vi "输入数据解析.vi"(0 "单个参数补充":dbl, 1 "从板号":dbl=1.0, 2 "主板二维码":string="BNET01", 3 "从板二维码":string="BNET01", 5 "主板引用":refnum<vi>, 7 "从板引用":refnum<vi>, 9 "主板选项":string="三级故障阀值", 11 "枚举":enum16{"主板", "从板"}(ring), 12 "快换":bool caption="快换写入") -> (4 "输出数组":dbl[][](array[numeric]), 6 "数组长度":dbl[](array[numeric]), 8 "循环次数":i32, 10 "命令":u32, 14 "名称":string[](array[string]), 15 "命令序号":u32[](array[numeric]))   [LabVIEW 2013] (continued)
                    n3519 = call "输入分辨率计算-EV05.vi"("1字节?"=TRUE, "数值"=w9118, "偏移量"=-40.0, "分辨率"=1.0) -> ("高字节1"=w9121:dbl)  [unwired: 1 in, 6 out]
                  }
                  frame Enabled {
                  }
                }
                n3520 = Build Array(w9117) -> (w9116:i32[])
              }
              frame 4 {
                # "整组温度不均衡"
                n3521 = disable-structure shown="启用" {
                  disable-tunnel: [w9131 255 ("高字节1")] -> w9127
                  disable-tunnel: w9125 -> [w9129 _]
                  frame Disabled {
                    n3522 = Unbundle By Name(w9129) -> ("整组温度不均衡"=w9128:dbl)
                    n3523 = call "输入分辨率计算-EV05.vi"("1字节?"=TRUE, "数值"=w9128, "偏移量"=0.0, "分辨率"=1.0) -> ("高字节1"=w9131:dbl)  [unwired: 1 in, 6 out]
                  }
                  frame Enabled {
                  }
                }
                n3524 = Build Array(w9127) -> (w9126:i32[])
              }
              frame 5 {
                # "单组电压不均衡"
                n3525 = disable-structure shown="启用" {
                  disable-tunnel: [w9143 w9146] -> w9138
                  disable-tunnel: [w9141 w9146] -> w9136
                  disable-tunnel: w9135 -> [w9140 _]
                  frame Disabled {
                    n3526 = Unbundle By Name(w9140) -> ("单组电压不均衡"=w9139:dbl)
                    n3527 = call "输入分辨率计算-EV05.vi"("1字节?"=FALSE, "数值"=w9139, "偏移量"=0.0, "分辨率"=0.001) -> ("低字节"=w9141:dbl, "高字节1"=w9143:dbl)  [unwired: 1 in, 5 out]
                  }
                  frame Enabled {
                    w9146 = 255 ("高字节1")
                  }
                }
                n3528 = Build Array(w9138, w9136) -> (w9137:i32[])
              }
              frame 6 {
                # "整组电压不均衡"
                n3529 = disable-structure shown="启用" {
                  disable-tunnel: [w9155 w9158] -> w9150
                  disable-tunnel: [w9153 w9158] -> w9148
                  disable-tunnel: w9147 -> [w9152 _]
                  frame Disabled {
                    n3530 = Unbundle By Name(w9152) -> ("整组电压不均衡"=w9151:dbl)
                    n3531 = call "输入分辨率计算-EV05.vi"("1字节?"=FALSE, "数值"=w9151, "偏移量"=0.0, "分辨率"=0.001) -> ("低字节"=w9153:dbl, "高字节1"=w9155:dbl)  [unwired: 1 in, 5 out]
                  }
                  frame Enabled {
                    w9158 = 255 ("高字节1")
                  }
                }
                n3532 = Build Array(w9150, w9148) -> (w9149:i32[])
              }
              frame 7 {
                # "单体电压过高"
                n3533 = disable-structure shown="启用" {
                  disable-tunnel: [w9167 w9170] -> w9162
                  disable-tunnel: [w9165 w9170] -> w9160
                  disable-tunnel: w9159 -> [w9164 _]
                  frame Disabled {
                    n3534 = Unbundle By Name(w9164) -> ("单体电压过高"=w9163:dbl)
                    n3535 = call "输入分辨率计算-EV05.vi"("1字节?"=FALSE, "数值"=w9163, "偏移量"=0.0, "分辨率"=0.001) -> ("低字节"=w9165:dbl, "高字节1"=w9167:dbl)  [unwired: 1 in, 5 out]
                  }
                  frame Enabled {
                    w9170 = 255 ("高字节1")
                  }
                }
                n3536 = Build Array(w9162, w9160) -> (w9161:i32[])
              }
              frame 8 {
                # "单体电压过低"
                n3537 = disable-structure shown="启用" {
                  disable-tunnel: [w9179 w9182] -> w9174
                  disable-tunnel: [w9177 w9182] -> w9172
                  disable-tunnel: w9171 -> [w9176 _]
                  frame Disabled {
                    n3538 = Unbundle By Name(w9176) -> ("单体电压过低"=w9175:dbl)
                    n3539 = call "输入分辨率计算-EV05.vi"("1字节?"=FALSE, "数值"=w9175, "偏移量"=0.0, "分辨率"=0.001) -> ("低字节"=w9177:dbl, "高字节1"=w9179:dbl)  [unwired: 1 in, 5 out]
                  }
                  frame Enabled {
                    w9182 = 255 ("高字节1")
                  }
                }
                n3540 = Build Array(w9174, w9172) -> (w9173:i32[])
              }
              frame 9 {
                # "充电电流过高"
                n3541 = disable-structure shown="启用" {
                  disable-tunnel: [w9191 w9194] -> w9186
                  disable-tunnel: [w9189 w9194] -> w9184
                  disable-tunnel: w9183 -> [w9188 _]
                  frame Disabled {
                    n3542 = Unbundle By Name(w9188) -> ("充电电流过高"=w9187:dbl)
                    n3543 = call "输入分辨率计算-EV05.vi"("1字节?"=FALSE, "数值"=w9187, "偏移量"=-3000.0, "分辨率"=0.1) -> ("低字节"=w9189:dbl, "高字节1"=w9191:dbl)  [unwired: 1 in, 5 out]
                  }
                  frame Enabled {
                    w9194 = 255 ("高字节1")
                  }
                }
                n3544 = Build Array(w9186, w9184) -> (w9185:i32[])
              }
              frame 10 {
                # "放电电流过高"
                n3545 = disable-structure shown="启用" {
                  disable-tunnel: [w9203 w9206] -> w9198
                  disable-tunnel: [w9201 w9206] -> w9196
                  disable-tunnel: w9195 -> [w9200 _]
                  frame Disabled {
                    n3546 = Unbundle By Name(w9200) -> ("放电电流过高"=w9199:dbl)
                    n3547 = call "输入分辨率计算-EV05.vi"("1字节?"=FALSE, "数值"=w9199, "偏移量"=-3000.0, "分辨率"=0.1) -> ("低字节"=w9201:dbl, "高字节1"=w9203:dbl)  [unwired: 1 in, 5 out]
                  }
                  frame Enabled {
                    w9206 = 255 ("高字节1")
                  }
                }
                n3548 = Build Array(w9198, w9196) -> (w9197:i32[])
              }
              frame 11 {
                # "单组温度不均衡"
                n3549 = disable-structure shown="启用" {
                  disable-tunnel: [w9212 255 ("高字节1")] -> w9209
                  disable-tunnel: w9207 -> [w9211 _]
                  frame Enabled {
                    n3550 = Unbundle By Name(w9211) -> ("单组温度不均衡"=w9210:dbl)
                    n3551 = call "输入分辨率计算-EV05.vi"("1字节?"=TRUE, "数值"=w9210, "分辨率"=1.0) -> ("高字节1"=w9212:dbl)  [unwired: 2 in, 6 out]
                  }
                  frame Disabled {
                  }
                }
                n3552 = Build Array(w9209) -> (w9208:dbl[])
              }
              frame 12 {
                # "SOC过高"
                n3553 = Unbundle By Name(w9220) -> ("SOC过高"=w9219:dbl)
                n3554 = call "输入分辨率计算-EV05.vi"("1字节?"=FALSE, "数值"=w9219, "偏移量"=0.0, "分辨率"=0.1) -> ("低字节"=w9221:dbl, "高字节1"=w9222:dbl)  [unwired: 1 in, 5 out]
                n3555 = call "二进制解析-8.6.vi"("索引"=4, "数值"=w9222) -> ("低位子数组"=w9225:i32[])  [unwired: 3 out]
                n3556 = call "二进制解析-8.6.vi"("索引"=4, "数值"=w9221) -> ("低位子数组"=w9217:i32[], "高位子数组"=w9224:i32[])  [unwired: 2 out]
                n3557 = Insert Into Array(array=w9225, new element=w9224) -> (w9223:i32[])  [unwired: 1 in]
                n3558 = call "数值二进制转十进制-8.6.vi"("子数组"=w9223) -> ("十进制数值"=w9218:i32)  [unwired: 4 out]
                n3559 = disable-structure shown="启用" {
                  disable-tunnel: w9218 -> [w9233 _]
                  disable-tunnel: [w9233 255 ("高字节1")] -> w9216
                  disable-tunnel: w9217 -> [w9232 _]
                  disable-tunnel: [w9232 i32[] [] ("低位子数组 29")] -> _
                  frame Disabled {
                  }
                  frame Enabled {
                  }
                }
                n3560 = Build Array(w9216, w9216) -> (w9229:i32[])
              }
              frame 13 {
                # "SOC过低"
                n3561 = Unbundle By Name(w9241) -> ("SOC过低"=w9240:dbl)
                n3562 = call "输入分辨率计算-EV05.vi"("1字节?"=FALSE, "数值"=w9240, "偏移量"=0.0, "分辨率"=0.1) -> ("低字节"=w9238:dbl, "高字节1"=w9239:dbl)  [unwired: 1 in, 5 out]
                n3563 = call "二进制解析-8.6.vi"("索引"=4, "数值"=w9239) -> ("低位子数组"=w9237:i32[])  [unwired: 3 out]
                n3564 = disable-structure shown="启用" {
                  disable-tunnel: w9238 -> [w9248 _]
                  disable-tunnel: [w9248 255 ("高字节1")] -> w9236
                  disable-tunnel: w9237 -> [w9247 _]
                  disable-tunnel: [w9247 i32[] [] ("低位子数组")] -> _
                  frame Disabled {
                    (unwired) i32[] [] ("低位子数组 4")
                  }
                  frame Enabled {
                  }
                }
                n3565 = Build Array(w9236, w9236) -> (w9244:i32[])
              }
              frame 14 {
                # "内阻过大"
                n3566 = disable-structure shown="启用" {
                  disable-tunnel: w9253 -> [w9258 _]
                  disable-tunnel: [w9254 255 ("高字节1")] -> w9251
                  frame Disabled {
                    n3567 = Unbundle By Name(w9258) -> ("内阻过大"=w9257:dbl)
                    n3568 = call "输入分辨率计算-EV05.vi"("1字节?"=TRUE, "数值"=w9257, "分辨率"=0.1) -> ("高字节1"=w9254:dbl)  [unwired: 2 in, 6 out]
                  }
                  frame Enabled {
                  }
                }
                n3569 = Build Array(w9251) -> (w9252:i32[])
              }
              frame 15 {
                # "极柱温度过高"
                n3570 = disable-structure shown="启用" {
                  disable-tunnel: w9262 -> [w9268 _]
                  disable-tunnel: [w9264 255 ("高字节1")] -> w9260
                  frame Disabled {
                    n3571 = Unbundle By Name(w9268) -> ("极柱温度过高"=w9267:dbl)
                    n3572 = call "输入分辨率计算-EV05.vi"("1字节?"=TRUE, "数值"=w9267, "偏移量"=-40.0, "分辨率"=1.0) -> ("高字节1"=w9264:dbl)  [unwired: 1 in, 6 out]
                  }
                  frame Enabled {
                  }
                }
                n3573 = Build Array(w9260) -> (w9261:i32[])
              }
              frame 16 {
                # "SOH过低"
                n3574 = disable-structure shown="启用" {
                  disable-tunnel: [w9285 w9293] -> w9272
                  disable-tunnel: w9271 -> [w9282 _]
                  disable-tunnel: [w9274 w9293] -> w9270
                  frame Disabled {
                    n3575 = Unbundle By Name(w9282) -> ("SOH过低"=w9281:dbl)
                    n3576 = call "输入分辨率计算-EV05.vi"("1字节?"=FALSE, "数值"=w9281, "偏移量"=0.0, "分辨率"=0.1) -> ("低字节"=w9283:dbl, "高字节1"=w9284:dbl)  [unwired: 1 in, 5 out]
                    n3577 = call "二进制解析-8.6.vi"("索引"=4, "数值"=w9284) -> ("低位子数组"=w9287:i32[])  [unwired: 3 out]
                    n3578 = call "二进制解析-8.6.vi"("索引"=4, "数值"=w9283) -> ("低位子数组"=w9276:i32[], "高位子数组"=w9286:i32[])  [unwired: 2 out]
                    n3579 = call "二进制解析-8.6.vi"("索引"=4, "数值"=0) -> ("低位子数组"=w9277:i32[])  [unwired: 3 out]
                    n3580 = Insert Into Array(array=w9287, new element=w9286) -> (w9280:i32[])  [unwired: 1 in]
                    n3581 = Insert Into Array(array=w9276, new element=w9277) -> (w9275:i32[])  [unwired: 1 in]
                    n3582 = call "数值二进制转十进制-8.6.vi"("子数组"=w9280) -> ("十进制数值"=w9285:i32)  [unwired: 4 out]
                    n3583 = call "数值二进制转十进制-8.6.vi"("子数组"=w9275) -> ("十进制数值"=w9274:i32)  [unwired: 4 out]
                  }
                  frame Enabled {
                    w9293 = 255 ("高字节1")
                  }
                }
                n3584 = Build Array(w9272, w9270) -> (w9273:i32[])
              }
            }
            n3585 = Insert Into Array(array=w9079, new element=w9080) -> (w9078:dbl[])  [unwired: 1 in]
          }
          n3586 = Build Array(w9075) -> (w9074:dbl[][])
          n3587 = Build Array("三级故障阀值") -> (w9065:string[])
        }
        frame "内阻过大" {
          n3588 = Unbundle By Name(w9299) -> ("一级故障"=w9300:refnum<vi>)
          n3589 = property class="Clust (严格)"(reference=w9300) -> ("Value"=w9298:T4)  [unwired: 1 in, 2 out]
          n3590 = for {
            N: 17 -> [_]
            tunnel: w9298 -> [w9310]
            shift-right: [w9307] -> w9304
            shift-left: dbl[] [] -> [w9308]
            i -> [w9311]
            n3591 = case shown="13" w9311 {
              tunnel: w9310 -> [w9312 w9323 w9334 w9344 w9354 w9364 w9376 w9388 w9400 w9412 w9424 w9436 w9450 w9471 w9483 w9492 w9501]
              tunnel: [w9313 w9324 w9335 w9345 w9355 w9366 w9378 w9390 w9402 w9414 w9426 w9437 w9459 w9474 w9482 w9491 w9503] -> w9309
              frame 0, Default {
                # "总电压过高"
                n3592 = disable-structure shown="启用" {
                  disable-tunnel: [w9319 w9322] -> w9315
                  disable-tunnel: [w9318 w9322] -> w9314
                  disable-tunnel: w9312 -> [w9317 _]
                  frame Disabled {
                    n3593 = Unbundle By Name(w9317) -> ("总电压过高"=w9316:dbl)
                    n3594 = call "输入分辨率计算-EV05.vi"("1字节?"=FALSE, "数值"=w9316, "分辨率"=0.1) -> ("低字节"=w9319:dbl, "高字节1"=w9318:dbl)  [unwired: 2 in, 5 out]
                  }
                  frame Enabled {
                    w9322 = 255 ("高字节1")
                  }
                }
                n3595 = Build Array(w9314, w9315) -> (w9313:i32[])
              }
              frame 1 {
                # "总电压过低"
                n3596 = disable-structure shown="启用" {
                  disable-tunnel: [w9330 w9333] -> w9326
                  disable-tunnel: [w9329 w9333] -> w9325
                  disable-tunnel: w9323 -> [w9328 _]
                  frame Disabled {
                    n3597 = Unbundle By Name(w9328) -> ("总电压过低"=w9327:dbl)
                    n3598 = call "输入分辨率计算-EV05.vi"("1字节?"=FALSE, "数值"=w9327, "分辨率"=0.1) -> ("低字节"=w9330:dbl, "高字节1"=w9329:dbl)  [unwired: 2 in, 5 out]
                  }
                  frame Enabled {
                    w9333 = 255 ("高字节1")
                  }
                }
                n3599 = Build Array(w9325, w9326) -> (w9324:i32[])
              }
              frame 2 {
                # "温度过高"
                n3600 = disable-structure shown="启用" {
                  disable-tunnel: [w9340 255 ("高字节1")] -> w9336
                  disable-tunnel: w9334 -> [w9338 _]
                  frame Disabled {
                    n3601 = Unbundle By Name(w9338) -> ("温度过高"=w9337:dbl)
                    n3602 = call "输入分辨率计算-EV05.vi"("1字节?"=TRUE, "数值"=w9337, "偏移量"=-40.0, "分辨率"=1.0) -> ("高字节1"=w9340:dbl)  [unwired: 1 in, 6 out]
                  }
                  frame Enabled {
                  }
                }
                n3603 = Build Array(w9336) -> (w9335:i32[])
              }
              frame 3 {
                # "温度过低"
                n3604 = disable-structure shown="启用" {
                  disable-tunnel: [w9350 255 ("高字节1")] -> w9346
                  disable-tunnel: w9344 -> [w9348 _]
                  frame Disabled {
                    n3605 = Unbundle By Name(w9348) -> ("温度过低"=w9347:dbl)
                    n3606 = call "输入分辨率计算-EV05.vi"("1字节?"=TRUE, "数值"=w9347, "偏移量"=-40.0, "分辨率"=1.0) -> ("高字节1"=w9350:dbl)  [unwired: 1 in, 6 out]
                  }
                  frame Enabled {
                  }
                }
                n3607 = Build Array(w9346) -> (w9345:i32[])
              }
              frame 4 {
                # "整组温度不均衡"
                n3608 = disable-structure shown="启用" {
                  disable-tunnel: [w9360 255 ("高字节1")] -> w9356
                  disable-tunnel: w9354 -> [w9358 _]
                  frame Disabled {
                    n3609 = Unbundle By Name(w9358) -> ("整组温度不均衡"=w9357:dbl)
                    n3610 = call "输入分辨率计算-EV05.vi"("1字节?"=TRUE, "数值"=w9357, "偏移量"=0.0, "分辨率"=1.0) -> ("高字节1"=w9360:dbl)  [unwired: 1 in, 6 out]
                  }
                  frame Enabled {
                  }
                }
                n3611 = Build Array(w9356) -> (w9355:i32[])
              }
              frame 5 {
                # "单组电压不均衡"
                n3612 = disable-structure shown="启用" {
                  disable-tunnel: [w9372 w9375] -> w9367
                  disable-tunnel: [w9370 w9375] -> w9365
                  disable-tunnel: w9364 -> [w9369 _]
                  frame Disabled {
                    n3613 = Unbundle By Name(w9369) -> ("单组电压不均衡"=w9368:dbl)
                    n3614 = call "输入分辨率计算-EV05.vi"("1字节?"=FALSE, "数值"=w9368, "偏移量"=0.0, "分辨率"=0.001) -> ("低字节"=w9370:dbl, "高字节1"=w9372:dbl)  [unwired: 1 in, 5 out]
                  }
                  frame Enabled {
                    w9375 = 255 ("高字节1")
                  }
                }
                n3615 = Build Array(w9367, w9365) -> (w9366:i32[])
              }
              frame 6 {
                # "整组电压不均衡"
                n3616 = disable-structure shown="启用" {
                  disable-tunnel: [w9384 w9387] -> w9379
                  disable-tunnel: [w9382 w9387] -> w9377
                  disable-tunnel: w9376 -> [w9381 _]
                  frame Disabled {
                    n3617 = Unbundle By Name(w9381) -> ("整组电压不均衡"=w9380:dbl)
                    n3618 = call "输入分辨率计算-EV05.vi"("1字节?"=FALSE, "数值"=w9380, "偏移量"=0.0, "分辨率"=0.001) -> ("低字节"=w9382:dbl, "高字节1"=w9384:dbl)  [unwired: 1 in, 5 out]
                  }
                  frame Enabled {
                    w9387 = 255 ("高字节1")
                  }
                }
                n3619 = Build Array(w9379, w9377) -> (w9378:i32[])
              }
              frame 7 {
                # "单体电压过高"
                n3620 = disable-structure shown="启用" {
                  disable-tunnel: [w9396 w9399] -> w9391
                  disable-tunnel: [w9394 w9399] -> w9389
                  disable-tunnel: w9388 -> [w9393 _]
                  frame Disabled {
                    n3621 = Unbundle By Name(w9393) -> ("单体电压过高"=w9392:dbl)
                    n3622 = call "输入分辨率计算-EV05.vi"("1字节?"=FALSE, "数值"=w9392, "偏移量"=0.0, "分辨率"=0.001) -> ("低字节"=w9394:dbl, "高字节1"=w9396:dbl)  [unwired: 1 in, 5 out]
                  }
                  frame Enabled {
                    w9399 = 255 ("高字节1")
                  }
                }
                n3623 = Build Array(w9391, w9389) -> (w9390:i32[])
              }
              frame 8 {
                # "单体电压过低"
                n3624 = disable-structure shown="启用" {
                  disable-tunnel: [w9408 w9411] -> w9403
                  disable-tunnel: [w9406 w9411] -> w9401
                  disable-tunnel: w9400 -> [w9405 _]
                  frame Disabled {
                    n3625 = Unbundle By Name(w9405) -> ("单体电压过低"=w9404:dbl)
                    n3626 = call "输入分辨率计算-EV05.vi"("1字节?"=FALSE, "数值"=w9404, "偏移量"=0.0, "分辨率"=0.001) -> ("低字节"=w9406:dbl, "高字节1"=w9408:dbl)  [unwired: 1 in, 5 out]
                  }
                  frame Enabled {
                    w9411 = 255 ("高字节1")
                  }
                }
                n3627 = Build Array(w9403, w9401) -> (w9402:i32[])
              }
              frame 9 {
                # "充电电流过高"
                n3628 = disable-structure shown="启用" {
                  disable-tunnel: [w9420 w9423] -> w9415
                  disable-tunnel: [w9418 w9423] -> w9413
                  disable-tunnel: w9412 -> [w9417 _]
                  frame Disabled {
                    n3629 = Unbundle By Name(w9417) -> ("充电电流过高"=w9416:dbl)
                    n3630 = call "输入分辨率计算-EV05.vi"("1字节?"=FALSE, "数值"=w9416, "偏移量"=-3000.0, "分辨率"=0.1) -> ("低字节"=w9418:dbl, "高字节1"=w9420:dbl)  [unwired: 1 in, 5 out]
                  }
                  frame Enabled {
                    w9423 = 255 ("高字节1")
                  }
                }
                n3631 = Build Array(w9415, w9413) -> (w9414:i32[])
              }
              frame 10 {
                # "放电电流过高"
                n3632 = disable-structure shown="启用" {
                  disable-tunnel: [w9432 w9435] -> w9427
                  disable-tunnel: [w9430 w9435] -> w9425
                  disable-tunnel: w9424 -> [w9429 _]
                  frame Disabled {
                    n3633 = Unbundle By Name(w9429) -> ("放电电流过高"=w9428:dbl)
                    n3634 = call "输入分辨率计算-EV05.vi"("1字节?"=FALSE, "数值"=w9428, "偏移量"=-3000.0, "分辨率"=0.1) -> ("低字节"=w9430:dbl, "高字节1"=w9432:dbl)  [unwired: 1 in, 5 out]
                  }
                  frame Enabled {
                    w9435 = 255 ("高字节1")
                  }
                }
                n3635 = Build Array(w9427, w9425) -> (w9426:i32[])
              }
              frame 11 {
                # "单组温度不均衡"
                n3636 = disable-structure shown="启用" {
                  disable-tunnel: [w9442 255 ("高字节1")] -> w9438
                  disable-tunnel: w9436 -> [w9440 _]
                  frame Disabled {
                    n3637 = Unbundle By Name(w9440) -> ("单组温度不均衡"=w9439:dbl)
                    n3638 = call "输入分辨率计算-EV05.vi"("1字节?"=TRUE, "数值"=w9439, "偏移量"=0.0, "分辨率"=1.0) -> ("高字节1"=w9442:dbl)  [unwired: 1 in, 6 out]
                  }
                  frame Enabled {
                  }
                }
                n3639 = Build Array(w9438) -> (w9437:i32[])
              }
              frame 12 {
                # "SOC过高"
                n3640 = Unbundle By Name(w9450) -> ("SOC过高"=w9449:dbl)
                n3641 = call "输入分辨率计算-EV05.vi"("1字节?"=FALSE, "数值"=w9449, "偏移量"=0.0, "分辨率"=0.1) -> ("低字节"=w9451:dbl, "高字节1"=w9452:dbl)  [unwired: 1 in, 5 out]
                n3642 = call "二进制解析-8.6.vi"("索引"=4, "数值"=w9452) -> ("低位子数组"=w9455:i32[])  [unwired: 3 out]
                n3643 = call "二进制解析-8.6.vi"("索引"=4, "数值"=w9451) -> ("低位子数组"=w9447:i32[], "高位子数组"=w9454:i32[])  [unwired: 2 out]
                n3644 = Insert Into Array(array=w9455, new element=w9454) -> (w9453:i32[])  [unwired: 1 in]
                n3645 = call "数值二进制转十进制-8.6.vi"("子数组"=w9453) -> ("十进制数值"=w9448:i32)  [unwired: 4 out]
                n3646 = disable-structure shown="启用" {
                  disable-tunnel: w9448 -> [w9463 _]
                  disable-tunnel: [w9463 255 ("高字节1")] -> w9446
                  disable-tunnel: w9447 -> [w9462 _]
                  disable-tunnel: [w9462 i32[] [] ("低位子数组 29")] -> _
                  frame Disabled {
                  }
                  frame Enabled {
                  }
                }
                n3647 = Build Array(w9446, w9446) -> (w9459:i32[])
              }
              frame 13 {
                # "SOC过低"
                n3648 = Unbundle By Name(w9471) -> ("SOC过低"=w9470:dbl)
                n3649 = call "输入分辨率计算-EV05.vi"("1字节?"=FALSE, "数值"=w9470, "偏移量"=0.0, "分辨率"=0.1) -> ("低字节"=w9468:dbl, "高字节1"=w9469:dbl)  [unwired: 1 in, 5 out]
                n3650 = call "二进制解析-8.6.vi"("索引"=4, "数值"=w9469) -> ("低位子数组"=w9467:i32[])  [unwired: 3 out]
                n3651 = disable-structure shown="启用" {
                  disable-tunnel: w9468 -> [w9478 _]
                  disable-tunnel: [w9478 255 ("高字节1")] -> w9466
                  disable-tunnel: w9467 -> [w9477 _]
                  disable-tunnel: [w9477 i32[] [] ("低位子数组")] -> _
                  frame Disabled {
                    (unwired) i32[] [] ("低位子数组 4")
                  }
                  frame Enabled {
                  }
                }
                n3652 = Build Array(w9466, w9466) -> (w9474:i32[])
              }
              frame 14 {
                # "内阻过大"
                n3653 = disable-structure shown="启用" {
                  disable-tunnel: w9483 -> [w9488 _]
                  disable-tunnel: [w9484 255 ("高字节1")] -> w9481
                  frame Enabled {
                    n3654 = Unbundle By Name(w9488) -> ("内阻过大"=w9487:dbl)
                    n3655 = call "输入分辨率计算-EV05.vi"("1字节?"=TRUE, "数值"=w9487, "分辨率"=0.1) -> ("高字节1"=w9484:dbl)  [unwired: 2 in, 6 out]
                  }
                  frame Disabled {
                  }
                }
                n3656 = Build Array(w9481) -> (w9482:dbl[])
              }
              frame 15 {
                # "极柱温度过高"
                n3657 = disable-structure shown="启用" {
                  disable-tunnel: w9492 -> [w9498 _]
                  disable-tunnel: [w9494 255 ("高字节1")] -> w9490
                  frame Disabled {
                    n3658 = Unbundle By Name(w9498) -> ("极柱温度过高"=w9497:dbl)
                    n3659 = call "输入分辨率计算-EV05.vi"("1字节?"=TRUE, "数值"=w9497, "偏移量"=-40.0, "分辨率"=1.0) -> ("高字节1"=w9494:dbl)  [unwired: 1 in, 6 out]
                  }
                  frame Enabled {
                  }
                }
                n3660 = Build Array(w9490) -> (w9491:i32[])
              }
              frame 16 {
                # "SOH过低"
                n3661 = disable-structure shown="启用" {
                  disable-tunnel: [w9515 w9523] -> w9502
                  disable-tunnel: w9501 -> [w9512 _]
                  disable-tunnel: [w9504 w9523] -> w9500
                  frame Disabled {
                    n3662 = Unbundle By Name(w9512) -> ("SOH过低"=w9511:dbl)
                    n3663 = call "输入分辨率计算-EV05.vi"("1字节?"=FALSE, "数值"=w9511, "偏移量"=0.0, "分辨率"=0.1) -> ("低字节"=w9513:dbl, "高字节1"=w9514:dbl)  [unwired: 1 in, 5 out]
                    n3664 = call "二进制解析-8.6.vi"("索引"=4, "数值"=w9514) -> ("低位子数组"=w9517:i32[])  [unwired: 3 out]
                    n3665 = call "二进制解析-8.6.vi"("索引"=4, "数值"=w9513) -> ("低位子数组"=w9506:i32[], "高位子数组"=w9516:i32[])  [unwired: 2 out]
                    n3666 = call "二进制解析-8.6.vi"("索引"=4, "数值"=0) -> ("低位子数组"=w9507:i32[])  [unwired: 3 out]
                    n3667 = Insert Into Array(array=w9517, new element=w9516) -> (w9510:i32[])  [unwired: 1 in]
                    n3668 = Insert Into Array(array=w9506, new element=w9507) -> (w9505:i32[])  [unwired: 1 in]
                    n3669 = call "数值二进制转十进制-8.6.vi"("子数组"=w9510) -> ("十进制数值"=w9515:i32)  [unwired: 4 out]
                    n3670 = call "数值二进制转十进制-8.6.vi"("子数组"=w9505) -> ("十进制数值"=w9504:i32)  [unwired: 4 out]
                  }
                  frame Enabled {
                    w9523 = 255 ("高字节1")
                  }
                }
                n3671 = Build Array(w9502, w9500) -> (w9503:i32[])
              }
            }
            n3672 = Insert Into Array(array=w9308, new element=w9309) -> (w9307:dbl[])  [unwired: 1 in]
          }
          n3673 = Build Array(w9304) -> (w9303:dbl[][])
          n3674 = Build Array("一级故障阀值") -> (w9294:string[])
        }
        frame "内阻过大(2)" {
          n3675 = Unbundle By Name(w9529) -> ("一级故障 2"=w9530:refnum<vi>)
          n3676 = property class="Clust (严格)"(reference=w9530) -> ("Value"=w9528:T4)  [unwired: 1 in, 2 out]
          n3677 = for {
            N: 17 -> [_]
            tunnel: w9528 -> [w9540]
            shift-right: [w9537] -> w9534
            shift-left: dbl[] [] -> [w9538]
            i -> [w9541]
            n3678 = case shown="13" w9541 {
              tunnel: w9540 -> [w9542 w9553 w9564 w9574 w9584 w9594 w9606 w9618 w9630 w9642 w9654 w9666 w9680 w9701 w9713 w9722 w9731]
              tunnel: [w9543 w9554 w9565 w9575 w9585 w9596 w9608 w9620 w9632 w9644 w9656 w9667 w9689 w9704 w9712 w9721 w9733] -> w9539
              frame 0, Default {
                # "总电压过高"
                n3679 = disable-structure shown="启用" {
                  disable-tunnel: [w9549 w9552] -> w9545
                  disable-tunnel: [w9548 w9552] -> w9544
                  disable-tunnel: w9542 -> [w9547 _]
                  frame Disabled {
                    n3680 = Unbundle By Name(w9547) -> ("总电压过高"=w9546:dbl)
                    n3681 = call "输入分辨率计算-EV05.vi"("1字节?"=FALSE, "数值"=w9546, "分辨率"=0.1) -> ("低字节"=w9549:dbl, "高字节1"=w9548:dbl)  [unwired: 2 in, 5 out]
                  }
                  frame Enabled {
                    w9552 = 255 ("高字节1")
                  }
                }
                n3682 = Build Array(w9544, w9545) -> (w9543:i32[])
              }
              frame 1 {
                # "总电压过低"
                n3683 = disable-structure shown="启用" {
                  disable-tunnel: [w9560 w9563] -> w9556
                  disable-tunnel: [w9559 w9563] -> w9555
                  disable-tunnel: w9553 -> [w9558 _]
                  frame Disabled {
                    n3684 = Unbundle By Name(w9558) -> ("总电压过低"=w9557:dbl)
                    n3685 = call "输入分辨率计算-EV05.vi"("1字节?"=FALSE, "数值"=w9557, "分辨率"=0.1) -> ("低字节"=w9560:dbl, "高字节1"=w9559:dbl)  [unwired: 2 in, 5 out]
                  }
                  frame Enabled {
                    w9563 = 255 ("高字节1")
                  }
                }
                n3686 = Build Array(w9555, w9556) -> (w9554:i32[])
              }
              frame 2 {
                # "温度过高"
                n3687 = disable-structure shown="启用" {
                  disable-tunnel: [w9570 255 ("高字节1")] -> w9566
                  disable-tunnel: w9564 -> [w9568 _]
                  frame Disabled {
                    n3688 = Unbundle By Name(w9568) -> ("温度过高"=w9567:dbl)
                    n3689 = call "输入分辨率计算-EV05.vi"("1字节?"=TRUE, "数值"=w9567, "偏移量"=-40.0, "分辨率"=1.0) -> ("高字节1"=w9570:dbl)  [unwired: 1 in, 6 out]
                  }
                  frame Enabled {
                  }
                }
                n3690 = Build Array(w9566) -> (w9565:i32[])
              }
              frame 3 {
                # "温度过低"
                n3691 = disable-structure shown="启用" {
                  disable-tunnel: [w9580 255 ("高字节1")] -> w9576
                  disable-tunnel: w9574 -> [w9578 _]
                  frame Disabled {
                    n3692 = Unbundle By Name(w9578) -> ("温度过低"=w9577:dbl)
                    n3693 = call "输入分辨率计算-EV05.vi"("1字节?"=TRUE, "数值"=w9577, "偏移量"=-40.0, "分辨率"=1.0) -> ("高字节1"=w9580:dbl)  [unwired: 1 in, 6 out]
                  }
                  frame Enabled {
                  }
                }
                n3694 = Build Array(w9576) -> (w9575:i32[])
              }
              frame 4 {
                # "整组温度不均衡"
                n3695 = disable-structure shown="启用" {
                  disable-tunnel: [w9590 255 ("高字节1")] -> w9586
                  disable-tunnel: w9584 -> [w9588 _]
                  frame Disabled {
                    n3696 = Unbundle By Name(w9588) -> ("整组温度不均衡"=w9587:dbl)
                    n3697 = call "输入分辨率计算-EV05.vi"("1字节?"=TRUE, "数值"=w9587, "偏移量"=0.0, "分辨率"=1.0) -> ("高字节1"=w9590:dbl)  [unwired: 1 in, 6 out]
                  }
                  frame Enabled {
                  }
                }
                n3698 = Build Array(w9586) -> (w9585:i32[])
              }
              frame 5 {
                # "单组电压不均衡"
                n3699 = disable-structure shown="启用" {
                  disable-tunnel: [w9602 w9605] -> w9597
                  disable-tunnel: [w9600 w9605] -> w9595
                  disable-tunnel: w9594 -> [w9599 _]
                  frame Disabled {
                    n3700 = Unbundle By Name(w9599) -> ("单组电压不均衡"=w9598:dbl)
                    n3701 = call "输入分辨率计算-EV05.vi"("1字节?"=FALSE, "数值"=w9598, "偏移量"=0.0, "分辨率"=0.001) -> ("低字节"=w9600:dbl, "高字节1"=w9602:dbl)  [unwired: 1 in, 5 out]
                  }
                  frame Enabled {
                    w9605 = 255 ("高字节1")
                  }
                }
                n3702 = Build Array(w9597, w9595) -> (w9596:i32[])
              }
              frame 6 {
                # "整组电压不均衡"
                n3703 = disable-structure shown="启用" {
                  disable-tunnel: [w9614 w9617] -> w9609
                  disable-tunnel: [w9612 w9617] -> w9607
                  disable-tunnel: w9606 -> [w9611 _]
                  frame Disabled {
                    n3704 = Unbundle By Name(w9611) -> ("整组电压不均衡"=w9610:dbl)
                    n3705 = call "输入分辨率计算-EV05.vi"("1字节?"=FALSE, "数值"=w9610, "偏移量"=0.0, "分辨率"=0.001) -> ("低字节"=w9612:dbl, "高字节1"=w9614:dbl)  [unwired: 1 in, 5 out]
                  }
                  frame Enabled {
                    w9617 = 255 ("高字节1")
                  }
                }
                n3706 = Build Array(w9609, w9607) -> (w9608:i32[])
              }
              frame 7 {
                # "单体电压过高"
                n3707 = disable-structure shown="启用" {
                  disable-tunnel: [w9626 w9629] -> w9621
                  disable-tunnel: [w9624 w9629] -> w9619
                  disable-tunnel: w9618 -> [w9623 _]
                  frame Disabled {
                    n3708 = Unbundle By Name(w9623) -> ("单体电压过高"=w9622:dbl)
                    n3709 = call "输入分辨率计算-EV05.vi"("1字节?"=FALSE, "数值"=w9622, "偏移量"=0.0, "分辨率"=0.001) -> ("低字节"=w9624:dbl, "高字节1"=w9626:dbl)  [unwired: 1 in, 5 out]
                  }
                  frame Enabled {
                    w9629 = 255 ("高字节1")
                  }
                }
                n3710 = Build Array(w9621, w9619) -> (w9620:i32[])
              }
              frame 8 {
                # "单体电压过低"
                n3711 = disable-structure shown="启用" {
                  disable-tunnel: [w9638 w9641] -> w9633
                  disable-tunnel: [w9636 w9641] -> w9631
                  disable-tunnel: w9630 -> [w9635 _]
                  frame Disabled {
                    n3712 = Unbundle By Name(w9635) -> ("单体电压过低"=w9634:dbl)
                    n3713 = call "输入分辨率计算-EV05.vi"("1字节?"=FALSE, "数值"=w9634, "偏移量"=0.0, "分辨率"=0.001) -> ("低字节"=w9636:dbl, "高字节1"=w9638:dbl)  [unwired: 1 in, 5 out]
                  }
                  frame Enabled {
                    w9641 = 255 ("高字节1")
                  }
                }
                n3714 = Build Array(w9633, w9631) -> (w9632:i32[])
              }
              frame 9 {
                # "充电电流过高"
                n3715 = disable-structure shown="启用" {
                  disable-tunnel: [w9650 w9653] -> w9645
                  disable-tunnel: [w9648 w9653] -> w9643
                  disable-tunnel: w9642 -> [w9647 _]
                  frame Disabled {
                    n3716 = Unbundle By Name(w9647) -> ("充电电流过高"=w9646:dbl)
                    n3717 = call "输入分辨率计算-EV05.vi"("1字节?"=FALSE, "数值"=w9646, "偏移量"=-3000.0, "分辨率"=0.1) -> ("低字节"=w9648:dbl, "高字节1"=w9650:dbl)  [unwired: 1 in, 5 out]
                  }
                  frame Enabled {
                    w9653 = 255 ("高字节1")
                  }
                }
                n3718 = Build Array(w9645, w9643) -> (w9644:i32[])
              }
              frame 10 {
                # "放电电流过高"
                n3719 = disable-structure shown="启用" {
                  disable-tunnel: [w9662 w9665] -> w9657
                  disable-tunnel: [w9660 w9665] -> w9655
                  disable-tunnel: w9654 -> [w9659 _]
                  frame Disabled {
                    n3720 = Unbundle By Name(w9659) -> ("放电电流过高"=w9658:dbl)
                    n3721 = call "输入分辨率计算-EV05.vi"("1字节?"=FALSE, "数值"=w9658, "偏移量"=-3000.0, "分辨率"=0.1) -> ("低字节"=w9660:dbl, "高字节1"=w9662:dbl)  [unwired: 1 in, 5 out]
                  }
                  frame Enabled {
                    w9665 = 255 ("高字节1")
                  }
                }
                n3722 = Build Array(w9657, w9655) -> (w9656:i32[])
              }
              frame 11 {
                # "单组温度不均衡"
                n3723 = disable-structure shown="启用" {
                  disable-tunnel: [w9672 255 ("高字节1")] -> w9668
                  disable-tunnel: w9666 -> [w9670 _]
                  frame Disabled {
                    n3724 = Unbundle By Name(w9670) -> ("单组温度不均衡"=w9669:dbl)
                    n3725 = call "输入分辨率计算-EV05.vi"("1字节?"=TRUE, "数值"=w9669, "偏移量"=0.0, "分辨率"=1.0) -> ("高字节1"=w9672:dbl)  [unwired: 1 in, 6 out]
                  }
                  frame Enabled {
                  }
                }
                n3726 = Build Array(w9668) -> (w9667:i32[])
              }
              frame 12 {
                # "SOC过高"
                n3727 = Unbundle By Name(w9680) -> ("SOC过高"=w9679:dbl)
                n3728 = call "输入分辨率计算-EV05.vi"("1字节?"=FALSE, "数值"=w9679, "偏移量"=0.0, "分辨率"=0.1) -> ("低字节"=w9681:dbl, "高字节1"=w9682:dbl)  [unwired: 1 in, 5 out]
                n3729 = call "二进制解析-8.6.vi"("索引"=4, "数值"=w9682) -> ("低位子数组"=w9685:i32[])  [unwired: 3 out]
                n3730 = call "二进制解析-8.6.vi"("索引"=4, "数值"=w9681) -> ("低位子数组"=w9677:i32[], "高位子数组"=w9684:i32[])  [unwired: 2 out]
                n3731 = Insert Into Array(array=w9685, new element=w9684) -> (w9683:i32[])  [unwired: 1 in]
                n3732 = call "数值二进制转十进制-8.6.vi"("子数组"=w9683) -> ("十进制数值"=w9678:i32)  [unwired: 4 out]
                n3733 = disable-structure shown="启用" {
                  disable-tunnel: w9678 -> [w9693 _]
                  disable-tunnel: [w9693 255 ("高字节1")] -> w9676
                  disable-tunnel: w9677 -> [w9692 _]
                  disable-tunnel: [w9692 i32[] [] ("低位子数组 29")] -> _
                  frame Disabled {
                  }
                  frame Enabled {
                  }
                }
                n3734 = Build Array(w9676, w9676) -> (w9689:i32[])
              }
              frame 13 {
                # "SOC过低"
                n3735 = Unbundle By Name(w9701) -> ("SOC过低"=w9700:dbl)
                n3736 = call "输入分辨率计算-EV05.vi"("1字节?"=FALSE, "数值"=w9700, "偏移量"=0.0, "分辨率"=0.1) -> ("低字节"=w9698:dbl, "高字节1"=w9699:dbl)  [unwired: 1 in, 5 out]
                n3737 = call "二进制解析-8.6.vi"("索引"=4, "数值"=w9699) -> ("低位子数组"=w9697:i32[])  [unwired: 3 out]
                n3738 = disable-structure shown="启用" {
                  disable-tunnel: w9698 -> [w9708 _]
                  disable-tunnel: [w9708 255 ("高字节1")] -> w9696
                  disable-tunnel: w9697 -> [w9707 _]
                  disable-tunnel: [w9707 i32[] [] ("低位子数组")] -> _
                  frame Disabled {
                    (unwired) i32[] [] ("低位子数组 4")
                  }
                  frame Enabled {
                  }
                }
                n3739 = Build Array(w9696, w9696) -> (w9704:i32[])
              }
              frame 14 {
                # "内阻过大"
                n3740 = disable-structure shown="启用" {
                  disable-tunnel: w9713 -> [w9718 _]
                  disable-tunnel: [w9714 255 ("高字节1")] -> w9711
                  frame Enabled {
                    n3741 = Unbundle By Name(w9718) -> ("内阻过大"=w9717:dbl)
                    n3742 = call "输入分辨率计算-EV05.vi"("1字节?"=TRUE, "数值"=w9717, "分辨率"=0.1) -> ("高字节1"=w9714:dbl)  [unwired: 2 in, 6 out]
                  }
                  frame Disabled {
                  }
                }
                n3743 = Build Array(w9711) -> (w9712:dbl[])
              }
              frame 15 {
                # "极柱温度过高"
                n3744 = disable-structure shown="启用" {
                  disable-tunnel: w9722 -> [w9728 _]
                  disable-tunnel: [w9724 255 ("高字节1")] -> w9720
                  frame Disabled {
                    n3745 = Unbundle By Name(w9728) -> ("极柱温度过高"=w9727:dbl)
                    n3746 = call "输入分辨率计算-EV05.vi"("1字节?"=TRUE, "数值"=w9727, "偏移量"=-40.0, "分辨率"=1.0) -> ("高字节1"=w9724:dbl)  [unwired: 1 in, 6 out]
                  }
                  frame Enabled {
                  }
                }
                n3747 = Build Array(w9720) -> (w9721:i32[])
              }
              frame 16 {
                # "SOH过低"
                n3748 = disable-structure shown="启用" {
                  disable-tunnel: [w9745 w9753] -> w9732
                  disable-tunnel: w9731 -> [w9742 _]
                  disable-tunnel: [w9734 w9753] -> w9730
                  frame Disabled {
                    n3749 = Unbundle By Name(w9742) -> ("SOH过低"=w9741:dbl)
                    n3750 = call "输入分辨率计算-EV05.vi"("1字节?"=FALSE, "数值"=w9741, "偏移量"=0.0, "分辨率"=0.1) -> ("低字节"=w9743:dbl, "高字节1"=w9744:dbl)  [unwired: 1 in, 5 out]
                    n3751 = call "二进制解析-8.6.vi"("索引"=4, "数值"=w9744) -> ("低位子数组"=w9747:i32[])  [unwired: 3 out]
                    n3752 = call "二进制解析-8.6.vi"("索引"=4, "数值"=w9743) -> ("低位子数组"=w9736:i32[], "高位子数组"=w9746:i32[])  [unwired: 2 out]
                    n3753 = call "二进制解析-8.6.vi"("索引"=4, "数值"=0) -> ("低位子数组"=w9737:i32[])  [unwired: 3 out]
                    n3754 = Insert Into Array(array=w9747, new element=w9746) -> (w9740:i32[])  [unwired: 1 in]
                    n3755 = Insert Into Array(array=w9736, new element=w9737) -> (w9735:i32[])  [unwired: 1 in]
                    n3756 = call "数值二进制转十进制-8.6.vi"("子数组"=w9740) -> ("十进制数值"=w9745:i32)  [unwired: 4 out]
                    n3757 = call "数值二进制转十进制-8.6.vi"("子数组"=w9735) -> ("十进制数值"=w9734:i32)  [unwired: 4 out]
                  }
                  frame Enabled {
                    w9753 = 255 ("高字节1")
                  }
                }
                n3758 = Build Array(w9732, w9730) -> (w9733:i32[])
              }
            }
            n3759 = Insert Into Array(array=w9538, new element=w9539) -> (w9537:dbl[])  [unwired: 1 in]
          }
          n3760 = Build Array(w9534) -> (w9533:dbl[][])
          n3761 = Build Array("二级故障阀值") -> (w9524:string[])
        }
        frame "内阻过大(3)" {
          n3762 = Unbundle By Name(w9759) -> ("一级故障 3"=w9760:refnum<vi>)
          n3763 = property class="Clust (严格)"(reference=w9760) -> ("Value"=w9758:T4)  [unwired: 1 in, 2 out]
          n3764 = for {
            N: 17 -> [_]
            tunnel: w9758 -> [w9770]
            shift-right: [w9767] -> w9764
            shift-left: dbl[] [] -> [w9768]
            i -> [w9771]
            n3765 = case shown="13" w9771 {
              tunnel: w9770 -> [w9772 w9783 w9794 w9804 w9814 w9824 w9836 w9848 w9860 w9872 w9884 w9896 w9910 w9931 w9943 w9952 w9961]
              tunnel: [w9773 w9784 w9795 w9805 w9815 w9826 w9838 w9850 w9862 w9874 w9886 w9897 w9919 w9934 w9942 w9951 w9963] -> w9769
              frame 0, Default {
                # "总电压过高"
                n3766 = disable-structure shown="启用" {
                  disable-tunnel: [w9779 w9782] -> w9775
                  disable-tunnel: [w9778 w9782] -> w9774
                  disable-tunnel: w9772 -> [w9777 _]
                  frame Disabled {
                    n3767 = Unbundle By Name(w9777) -> ("总电压过高"=w9776:dbl)
                    n3768 = call "输入分辨率计算-EV05.vi"("1字节?"=FALSE, "数值"=w9776, "分辨率"=0.1) -> ("低字节"=w9779:dbl, "高字节1"=w9778:dbl)  [unwired: 2 in, 5 out]
                  }
                  frame Enabled {
                    w9782 = 255 ("高字节1")
                  }
                }
                n3769 = Build Array(w9774, w9775) -> (w9773:i32[])
              }
              frame 1 {
                # "总电压过低"
                n3770 = disable-structure shown="启用" {
                  disable-tunnel: [w9790 w9793] -> w9786
                  disable-tunnel: [w9789 w9793] -> w9785
                  disable-tunnel: w9783 -> [w9788 _]
                  frame Disabled {
                    n3771 = Unbundle By Name(w9788) -> ("总电压过低"=w9787:dbl)
                    n3772 = call "输入分辨率计算-EV05.vi"("1字节?"=FALSE, "数值"=w9787, "分辨率"=0.1) -> ("低字节"=w9790:dbl, "高字节1"=w9789:dbl)  [unwired: 2 in, 5 out]
                  }
                  frame Enabled {
                    w9793 = 255 ("高字节1")
                  }
                }
                n3773 = Build Array(w9785, w9786) -> (w9784:i32[])
              }
              frame 2 {
                # "温度过高"
                n3774 = disable-structure shown="启用" {
                  disable-tunnel: [w9800 255 ("高字节1")] -> w9796
                  disable-tunnel: w9794 -> [w9798 _]
                  frame Disabled {
                    n3775 = Unbundle By Name(w9798) -> ("温度过高"=w9797:dbl)
                    n3776 = call "输入分辨率计算-EV05.vi"("1字节?"=TRUE, "数值"=w9797, "偏移量"=-40.0, "分辨率"=1.0) -> ("高字节1"=w9800:dbl)  [unwired: 1 in, 6 out]
                  }
                  frame Enabled {
                  }
                }
                n3777 = Build Array(w9796) -> (w9795:i32[])
              }
              frame 3 {
                # "温度过低"
                n3778 = disable-structure shown="启用" {
                  disable-tunnel: [w9810 255 ("高字节1")] -> w9806
                  disable-tunnel: w9804 -> [w9808 _]
                  frame Disabled {
                    n3779 = Unbundle By Name(w9808) -> ("温度过低"=w9807:dbl)
                    n3780 = call "输入分辨率计算-EV05.vi"("1字节?"=TRUE, "数值"=w9807, "偏移量"=-40.0, "分辨率"=1.0) -> ("高字节1"=w9810:dbl)  [unwired: 1 in, 6 out]
                  }
                  frame Enabled {
                  }
                }
                n3781 = Build Array(w9806) -> (w9805:i32[])
              }
              frame 4 {
                # "整组温度不均衡"
                n3782 = disable-structure shown="启用" {
                  disable-tunnel: [w9820 255 ("高字节1")] -> w9816
                  disable-tunnel: w9814 -> [w9818 _]
                  frame Disabled {
                    n3783 = Unbundle By Name(w9818) -> ("整组温度不均衡"=w9817:dbl)
                    n3784 = call "输入分辨率计算-EV05.vi"("1字节?"=TRUE, "数值"=w9817, "偏移量"=0.0, "分辨率"=1.0) -> ("高字节1"=w9820:dbl)  [unwired: 1 in, 6 out]
                  }
                  frame Enabled {
                  }
                }
                n3785 = Build Array(w9816) -> (w9815:i32[])
              }
              frame 5 {
                # "单组电压不均衡"
                n3786 = disable-structure shown="启用" {
                  disable-tunnel: [w9832 w9835] -> w9827
                  disable-tunnel: [w9830 w9835] -> w9825
                  disable-tunnel: w9824 -> [w9829 _]
                  frame Disabled {
                    n3787 = Unbundle By Name(w9829) -> ("单组电压不均衡"=w9828:dbl)
                    n3788 = call "输入分辨率计算-EV05.vi"("1字节?"=FALSE, "数值"=w9828, "偏移量"=0.0, "分辨率"=0.001) -> ("低字节"=w9830:dbl, "高字节1"=w9832:dbl)  [unwired: 1 in, 5 out]
                  }
                  frame Enabled {
                    w9835 = 255 ("高字节1")
                  }
                }
                n3789 = Build Array(w9827, w9825) -> (w9826:i32[])
              }
              frame 6 {
                # "整组电压不均衡"
                n3790 = disable-structure shown="启用" {
                  disable-tunnel: [w9844 w9847] -> w9839
                  disable-tunnel: [w9842 w9847] -> w9837
                  disable-tunnel: w9836 -> [w9841 _]
                  frame Disabled {
                    n3791 = Unbundle By Name(w9841) -> ("整组电压不均衡"=w9840:dbl)
                    n3792 = call "输入分辨率计算-EV05.vi"("1字节?"=FALSE, "数值"=w9840, "偏移量"=0.0, "分辨率"=0.001) -> ("低字节"=w9842:dbl, "高字节1"=w9844:dbl)  [unwired: 1 in, 5 out]
                  }
                  frame Enabled {
                    w9847 = 255 ("高字节1")
                  }
                }
                n3793 = Build Array(w9839, w9837) -> (w9838:i32[])
              }
              frame 7 {
                # "单体电压过高"
                n3794 = disable-structure shown="启用" {
                  disable-tunnel: [w9856 w9859] -> w9851
                  disable-tunnel: [w9854 w9859] -> w9849
                  disable-tunnel: w9848 -> [w9853 _]
                  frame Disabled {
                    n3795 = Unbundle By Name(w9853) -> ("单体电压过高"=w9852:dbl)
                    n3796 = call "输入分辨率计算-EV05.vi"("1字节?"=FALSE, "数值"=w9852, "偏移量"=0.0, "分辨率"=0.001) -> ("低字节"=w9854:dbl, "高字节1"=w9856:dbl)  [unwired: 1 in, 5 out]
                  }
                  frame Enabled {
                    w9859 = 255 ("高字节1")
                  }
                }
                n3797 = Build Array(w9851, w9849) -> (w9850:i32[])
              }
              frame 8 {
                # "单体电压过低"
                n3798 = disable-structure shown="启用" {
                  disable-tunnel: [w9868 w9871] -> w9863
                  disable-tunnel: [w9866 w9871] -> w9861
                  disable-tunnel: w9860 -> [w9865 _]
                  frame Disabled {
                    n3799 = Unbundle By Name(w9865) -> ("单体电压过低"=w9864:dbl)
                    n3800 = call "输入分辨率计算-EV05.vi"("1字节?"=FALSE, "数值"=w9864, "偏移量"=0.0, "分辨率"=0.001) -> ("低字节"=w9866:dbl, "高字节1"=w9868:dbl)  [unwired: 1 in, 5 out]
                  }
                  frame Enabled {
                    w9871 = 255 ("高字节1")
                  }
                }
                n3801 = Build Array(w9863, w9861) -> (w9862:i32[])
              }
              frame 9 {
                # "充电电流过高"
                n3802 = disable-structure shown="启用" {
                  disable-tunnel: [w9880 w9883] -> w9875
                  disable-tunnel: [w9878 w9883] -> w9873
                  disable-tunnel: w9872 -> [w9877 _]
                  frame Disabled {
                    n3803 = Unbundle By Name(w9877) -> ("充电电流过高"=w9876:dbl)
                    n3804 = call "输入分辨率计算-EV05.vi"("1字节?"=FALSE, "数值"=w9876, "偏移量"=-3000.0, "分辨率"=0.1) -> ("低字节"=w9878:dbl, "高字节1"=w9880:dbl)  [unwired: 1 in, 5 out]
                  }
                  frame Enabled {
                    w9883 = 255 ("高字节1")
                  }
                }
                n3805 = Build Array(w9875, w9873) -> (w9874:i32[])
              }
              frame 10 {
                # "放电电流过高"
                n3806 = disable-structure shown="启用" {
                  disable-tunnel: [w9892 w9895] -> w9887
                  disable-tunnel: [w9890 w9895] -> w9885
                  disable-tunnel: w9884 -> [w9889 _]
                  frame Disabled {
                    n3807 = Unbundle By Name(w9889) -> ("放电电流过高"=w9888:dbl)
                    n3808 = call "输入分辨率计算-EV05.vi"("1字节?"=FALSE, "数值"=w9888, "偏移量"=-3000.0, "分辨率"=0.1) -> ("低字节"=w9890:dbl, "高字节1"=w9892:dbl)  [unwired: 1 in, 5 out]
                  }
                  frame Enabled {
                    w9895 = 255 ("高字节1")
                  }
                }
                n3809 = Build Array(w9887, w9885) -> (w9886:i32[])
              }
              frame 11 {
                # "单组温度不均衡"
                n3810 = disable-structure shown="启用" {
                  disable-tunnel: [w9902 255 ("高字节1")] -> w9898
                  disable-tunnel: w9896 -> [w9900 _]
                  frame Disabled {
                    n3811 = Unbundle By Name(w9900) -> ("单组温度不均衡"=w9899:dbl)
                    n3812 = call "输入分辨率计算-EV05.vi"("1字节?"=TRUE, "数值"=w9899, "偏移量"=0.0, "分辨率"=1.0) -> ("高字节1"=w9902:dbl)  [unwired: 1 in, 6 out]
                  }
                  frame Enabled {
                  }
                }
                n3813 = Build Array(w9898) -> (w9897:i32[])
              }
              frame 12 {
                # "SOC过高"
                n3814 = Unbundle By Name(w9910) -> ("SOC过高"=w9909:dbl)
                n3815 = call "输入分辨率计算-EV05.vi"("1字节?"=FALSE, "数值"=w9909, "偏移量"=0.0, "分辨率"=0.1) -> ("低字节"=w9911:dbl, "高字节1"=w9912:dbl)  [unwired: 1 in, 5 out]
                n3816 = call "二进制解析-8.6.vi"("索引"=4, "数值"=w9912) -> ("低位子数组"=w9915:i32[])  [unwired: 3 out]
                n3817 = call "二进制解析-8.6.vi"("索引"=4, "数值"=w9911) -> ("低位子数组"=w9907:i32[], "高位子数组"=w9914:i32[])  [unwired: 2 out]
                n3818 = Insert Into Array(array=w9915, new element=w9914) -> (w9913:i32[])  [unwired: 1 in]
                n3819 = call "数值二进制转十进制-8.6.vi"("子数组"=w9913) -> ("十进制数值"=w9908:i32)  [unwired: 4 out]
                n3820 = disable-structure shown="启用" {
                  disable-tunnel: w9908 -> [w9923 _]
                  disable-tunnel: [w9923 255 ("高字节1")] -> w9906
                  disable-tunnel: w9907 -> [w9922 _]
                  disable-tunnel: [w9922 i32[] [] ("低位子数组 29")] -> _
                  frame Disabled {
                  }
                  frame Enabled {
                  }
                }
                n3821 = Build Array(w9906, w9906) -> (w9919:i32[])
              }
              frame 13 {
                # "SOC过低"
                n3822 = Unbundle By Name(w9931) -> ("SOC过低"=w9930:dbl)
                n3823 = call "输入分辨率计算-EV05.vi"("1字节?"=FALSE, "数值"=w9930, "偏移量"=0.0, "分辨率"=0.1) -> ("低字节"=w9928:dbl, "高字节1"=w9929:dbl)  [unwired: 1 in, 5 out]
                n3824 = call "二进制解析-8.6.vi"("索引"=4, "数值"=w9929) -> ("低位子数组"=w9927:i32[])  [unwired: 3 out]
                n3825 = disable-structure shown="启用" {
                  disable-tunnel: w9928 -> [w9938 _]
                  disable-tunnel: [w9938 255 ("高字节1")] -> w9926
                  disable-tunnel: w9927 -> [w9937 _]
                  disable-tunnel: [w9937 i32[] [] ("低位子数组")] -> _
                  frame Disabled {
                    (unwired) i32[] [] ("低位子数组 4")
                  }
                  frame Enabled {
                  }
                }
                n3826 = Build Array(w9926, w9926) -> (w9934:i32[])
              }
              frame 14 {
                # "内阻过大"
                n3827 = disable-structure shown="启用" {
                  disable-tunnel: w9943 -> [w9948 _]
                  disable-tunnel: [w9944 255 ("高字节1")] -> w9941
                  frame Enabled {
                    n3828 = Unbundle By Name(w9948) -> ("内阻过大"=w9947:dbl)
                    n3829 = call "输入分辨率计算-EV05.vi"("1字节?"=TRUE, "数值"=w9947, "分辨率"=0.1) -> ("高字节1"=w9944:dbl)  [unwired: 2 in, 6 out]
                  }
                  frame Disabled {
                  }
                }
                n3830 = Build Array(w9941) -> (w9942:dbl[])
              }
              frame 15 {
